vi "CameraConnect.vi"(8 "error in (no error)":errorcluster, 9 "serial":u64 caption="Serial number:" format="%x", 10 "name":string caption="Connecting to camera:", 11 "NIvision in":refnum<class "IMAQdx.lvclass">) -> (0 "error out":errorcluster, 2 "CameraInfo":T1 {"serial" format="%x"}, 3 "NIvision out":refnum<class "IMAQdx.lvclass">)   [LabVIEW 2010, in "IMAQdx.lvclass"]
doc: "Creates an instance of the class, connected to a device with the specified serial number"
uses:
  IMAQdx.lvclass
  CameraBase/CameraInfo.ctl
  <vilib>/vision/driver/IMAQdx.llb/IMAQdx Acquisition Mode.ctl
  IMAQdx.lvclass/IMAQdx.ctl
  CameraBase/CameraBase.lvclass
  <vilib>/vision/driver/NI_Vision_Acquisition_Software.lvlib
panel:
  # "IMAQdx"
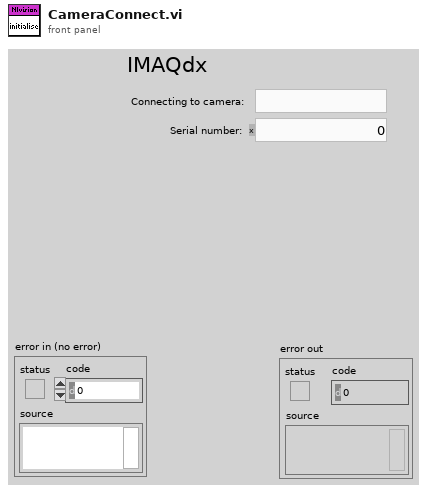
[diagram p1: front panel]
types:
  T1 = typedef "CameraInfo.ctl" = cluster{"name":string, "serial":u64, "interface":string, "make":string, "model":string, "pixel_w":dbl, "pixel_h":dbl}
  T2 = typedef "NI_Vision_Acquisition_Software.lvlib/IMAQdx Acquisition Mode.ctl" = enum32{"One Shot", "Continuous"}
  T3 = cluster{"Type":u32, "Version":u32, "Flags":u32, "SerialNumberHigh":u32, "SerialNumberLow":u32, "BusType":u32, "InterfaceName":string, "VendorName":string, "ModelName":string, "CameraFileName":string, "CameraAttributeURL":string}[]
  T4 = typedef "IMAQdx.ctl" = refnum<k21>
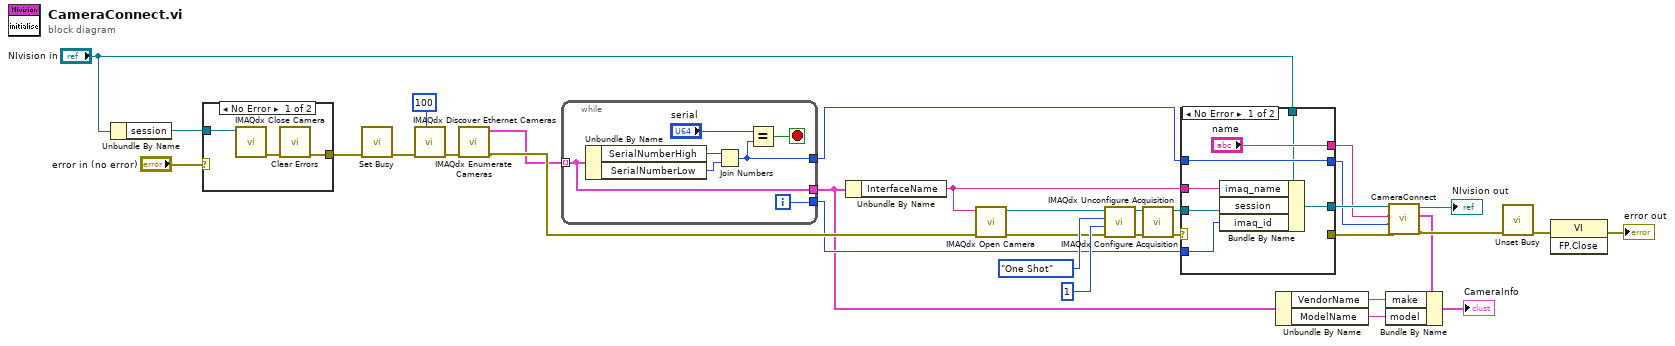
[diagram p0: block diagram]
diagram:
  n1 = Unbundle By Name("NIvision in") -> ("session"=w33:refnum<k21>)
  n2 = case shown="No Error" "error in (no error)" {
    selector: "error in (no error)" -> [_ w37]
    tunnel: [w34 w37] -> w31
    tunnel: w33 -> [w35 _]
    frame No Error {
      n3 = call <vilib>:"IMAQdx Close Camera.vi"("Session In"=w35) -> ("error out"=w36:errorcluster)  [unwired: 10 in]
      n4 = call <vilib>:"Clear Errors.vi"("error in (no error)"=w36) -> ("error out"=w34:errorcluster)  [unwired: 6 in]
    }
    frame Error {
    }
  }
  n5 = call <vilib>:"Set Busy.vi"("error in (no error)"=w31) -> ("error out"=w11:errorcluster)  [unwired: 9 in, 1 out]
  n6 = call <vilib>:"IMAQdx Discover Ethernet Cameras.vi"("Timeout (1000 ms)"=u32 100, "error in"=w11) -> ("error out"=w12:errorcluster)  [unwired: 9 in]
  n7 = call <vilib>:"IMAQdx Enumerate Cameras.vi"("error in"=w12) -> ("error out"=w10:errorcluster, "Camera Information Array"=w9:T3)  [unwired: 9 in]
  n8 = while {
    tunnel: w9 -> [w39] mode=indexing
    tunnel: [w40] -> w8
    tunnel: [w39] -> w3
    tunnel: [w38] -> w7
    i -> [w38]
    stop <- w44 stop-if-true
    n9 = Unbundle By Name(w39) -> ("SerialNumberHigh"=w41:u32, "SerialNumberLow"=w42:u32)
    n10 = Join Numbers(hi=w41, lo=w42) -> ((hi.lo)=w40:u64)
    n11 = Equal?(x="serial", y=w40) -> (x = y?=w44:bool)
  }
  n12 = Unbundle By Name(w3) -> ("InterfaceName"=w6:string)
  n13 = call <vilib>:"IMAQdx Open Camera.vi"("error in"=w10, "Session In"=w6) -> ("error out"=w16:errorcluster, "Session Out"=w29:T4)  [unwired: 8 in]
  n14 = call <vilib>:"IMAQdx Configure Acquisition.vi"("error in"=w16, "Number of Buffers"=u32 1, "Continuous?"=IMAQdx_Acquisition_Mode."One Shot", "Session In"=w29) -> ("error out"=w26:errorcluster, "Session Out"=w17:T4)  [unwired: 6 in]
  n15 = call <vilib>:"IMAQdx Unconfigure Acquisition.vi"("error in"=w26, "Session In"=w17) -> ("error out"=w24:errorcluster, "Session Out"=w25:T4)  [unwired: 8 in]
  n16 = case shown="No Error" w24 {
    selector: w24 -> [_ w53]
    tunnel: ["name" _] -> w20
    tunnel: w8 -> [w50 _]
    tunnel: [w50 _] -> w21
    tunnel: "NIvision in" -> [w49 w52]
    tunnel: w25 -> [w48 _]
    tunnel: w6 -> [w47 _]
    tunnel: w7 -> [w46 _]
    tunnel: [w45 w52] -> w23
    tunnel: [_ w53] -> w22
    frame No Error {
      n17 = Bundle By Name(cluster=w49, "imaq_name"=w47, "session"=w48, "imaq_id"=w46) -> (w45:refnum<class "IMAQdx.lvclass">)
    }
    frame Error {
    }
  }
  n18 = Unbundle By Name(w3) -> ("VendorName"=w2:string, "ModelName"=w1:string)
  n19 = call-parent "CameraConnect.vi"("error in (no error)"=w22, "serial"=w21, "name"=w20, "CameraBase in"=w23) -> ("error out"=w18:errorcluster, "CameraInfo"=w5:T1, "CameraBase out"=→"NIvision out":refnum<class "IMAQdx.lvclass">)  [unwired: 5 in]
  n20 = Bundle By Name(cluster=w5, "make"=w2, "model"=w1) -> (→"CameraInfo":T1)
  n21 = call <vilib>:"Unset Busy.vi"("error in (no error)"=w18) -> ("error out"=w15:errorcluster)  [unwired: 10 in]
  n22 = invoke class="VI" method="FP.Close"(error in=w15) -> (error out=→"error out":errorcluster)  [unwired: 2 in, 2 out]
